vi "proto_json.vi"() -> ()   [LabVIEW 2019]
uses:
  mmWave_driver_Py/LV-API/mmW_commands/TypeDefs/set_tx_freq.ctl
  <vilib>/addons/_JKI.lib/Serialization/JSON/JKI JSON Serialization.lvlib
  mmWave_driver_Py/LV-API/mmW_commands/mmW_commands.lvlib
panel:
  out "data":T1
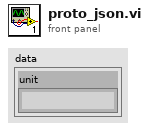
[diagram p1: front panel]
types:
  T1 = typedef "mmW_commands.lvlib/set_tx_freq.ctl" = cluster{"unit":string}
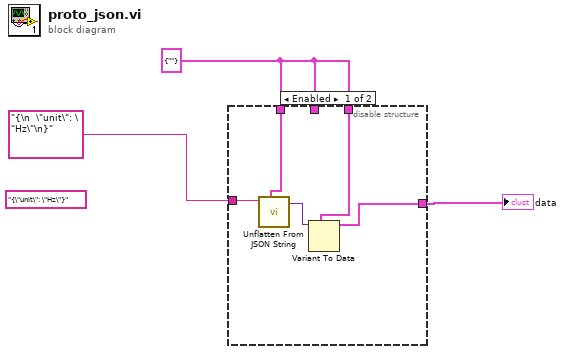
[diagram p0: block diagram]
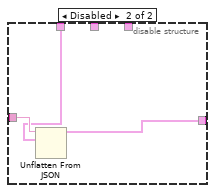
[diagram p2: hidden frame]
diagram:
  (unwired) "{\"unit\": \"Hz\"}" ("JSON String")
  w2 = T1 {"unit"=""}
  n1 = disable-structure shown="Enabled" {
    disable-tunnel: "{\n  \"unit\": \"Hz\"\n}" ("JSON String") -> [w8 w11]
    disable-tunnel: [w4 w9] -> w3
    disable-tunnel: w2 -> [w7 w10]
    disable-tunnel: w2 -> [_ _]
    disable-tunnel: w2 -> [w5 _]
    frame Enabled {
      n2 = call <vilib>:"Unflatten From JSON String.vi"("Type and Defaults"=w7, "JSON String"=w8) -> ("Variant"=w6:variant)  [unwired: 8 in, 1 out]
      n3 = Variant To Data(type=w5, Variant=w6) -> (data=w4:T1)  [unwired: 1 in, 1 out]
    }
    frame Disabled {
      n4 = Unflatten From JSON(JSON string=w11, type and defaults=w10) -> (value=w9:T1)  [unwired: 5 in, 1 out]
    }
  }
  "data" <- w3
